vi "WPI_SolenoidSafetyUpdate.vi"(8 "error in (no error)":errorcluster, 11 "SolenoidDevRef":T1={"DevStatus"={"status"=FALSE, "code"=0, "source"=""}, "Pneumatics Control Module"=1, "Forward Solenoid Channel"=enum."Solenoid 1", "Reverse Solenoid Channel"=enum."Invalid"}) -> (0 "error out":errorcluster, 3 "SolenoidDevRef 2":T1={"DevStatus"={"status"=FALSE, "code"=0, "source"=""}, "Pneumatics Control Module"=1, "Forward Solenoid Channel"=enum."Solenoid 1", "Reverse Solenoid Channel"=enum."Invalid"})   [LabVIEW 2017]
doc: "Updates the safety output for Solenoids. When Safety Ouput has been enabled, this VI must be called in a loop that is faster than the <B>timeout</B> value of Safety Config VI. Otherwise the Solenoid output will be suspended until the next time Solenoid is updated.\n\nThis software is licensed. Open the labview\\readme\\WPI Robotics Library Open Source License.txt file for more information."
uses:
  <vilib>/Rock Robotics/WPI/Solenoid/WPI_SolenoidDevRef.ctl
  <vilib>/Rock Robotics/WPI/Solenoid/WPI_SolenoidChannel.ctl
  <vilib>/Rock Robotics/WPI/SafetyOutput/WPI_SafetyOutputCheckMenu.ctl
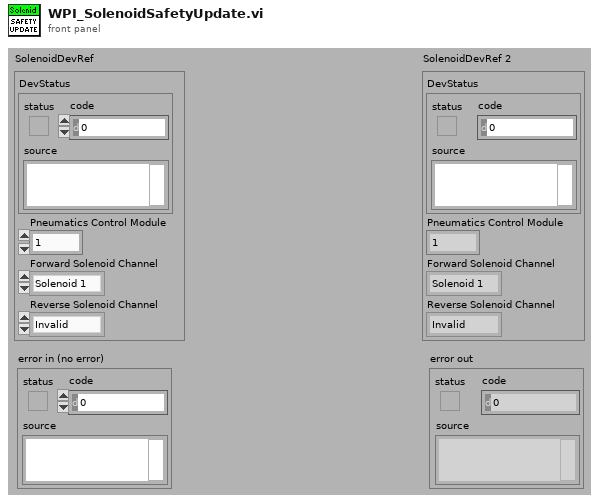
[diagram p1: front panel]
types:
  T1 = typedef "WPI_SolenoidDevRef.ctl" = cluster{"DevStatus":errorcluster, "Pneumatics Control Module":u8, "Forward Solenoid Channel":T2, "Reverse Solenoid Channel":T2}
  T2 = typedef "WPI_SolenoidChannel.ctl" = enum8{"Solenoid 0", "Solenoid 1", "Solenoid 2", "Solenoid 3", "Solenoid 4", "Solenoid 5", "Solenoid 6", "Solenoid 7", "Invalid"}
  T3 = typedef "WPI_SafetyOutputCheckMenu.ctl" = enum16{"test", "add", "remove", "update"}
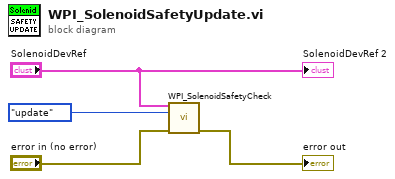
[diagram p0: block diagram]
diagram:
  n1 = call <vilib>:"WPI_SolenoidSafetyCheck.vi"("SolenoidDevRef"="SolenoidDevRef", "menu"=WPI_SafetyOutputCheckMenu."update", "error in (no error)"="error in (no error)") -> ("error out"=→"error out":errorcluster)  [unwired: 12 out]
  "SolenoidDevRef 2" <- "SolenoidDevRef"
